vi "ARCO Reactor Read Client.vi"() -> ()   [LabVIEW 2017]
uses:
  <vilib>/OPCUA/controls/NodeIds.ctl
  <vilib>/OPCUA/controls/NodeId.ctl
  <vilib>/OPCUA/NI OPC UA Client.lvlib
panel:
  in  "stop":bool
  out "error out":errorcluster
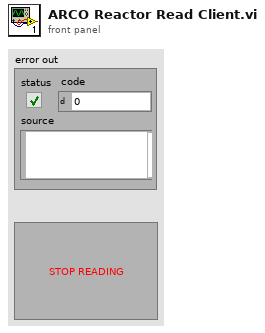
[diagram p1: front panel]
types:
  T1 = cluster{"message mode":enum16{"None", "Sign", "Sign and Encrypt"}, "security":enum16{"Basic256", "Basic128Rsa15"}}
  T2 = typedef "NodeIds.ctl" = T3[]
  T3 = typedef "NodeId.ctl" = string
  T4 = typedef "OPC UA Client Refnum.ctl" = refnum<k21>
  T5 = typedef "Subscription ID.ctl" = u32
  T6 = typedef "Subscription Data Change.ctl" = cluster{"node ID":T3, " value":variant, "timestamp":timestamp, "data type":T7, "status code":T8}
  T7 = typedef "Data Type.ctl" = u16
  T8 = typedef "OPC UA StatusCode.ctl" = u32
  T9 = cluster{"[0]":sgl, "[1]":sgl, "[2]":sgl, "[3]":sgl, "[4]":sgl, "[5]":sgl, "[6]":sgl, "[7]":sgl, "[8]":sgl, "[9]":sgl, "[10]":sgl, "[11]":sgl, "[12]":sgl, "[13]":sgl, "[14]":sgl, "[15]":sgl, "[16]":sgl, "[17]":sgl, "[18]":sgl, "[19]":sgl, "[20]":sgl, "[21]":sgl, "[22]":sgl, "[23]":sgl, "[24]":sgl, "[25]":sgl, "[26]":sgl, "[27]":sgl, "[28]":sgl, "[29]":sgl, "[30]":sgl, "[31]":sgl, "[32]":sgl, "[33]":sgl, "[34]":sgl, "[35]":sgl, "[36]":sgl, "[37]":sgl, "[38]":sgl, "[39]":sgl, "[40]":sgl, "[41]":sgl, "[42]":sgl, "[43]":sgl, "[44]":sgl, "[45]":sgl, "[46]":sgl, "[47]":sgl, "[48]":sgl, "[49]":sgl, "[50]":sgl, "[51]":sgl, "[52]":sgl, "[53]":sgl, "[54]":sgl, "[55]":sgl, "[56]":sgl}
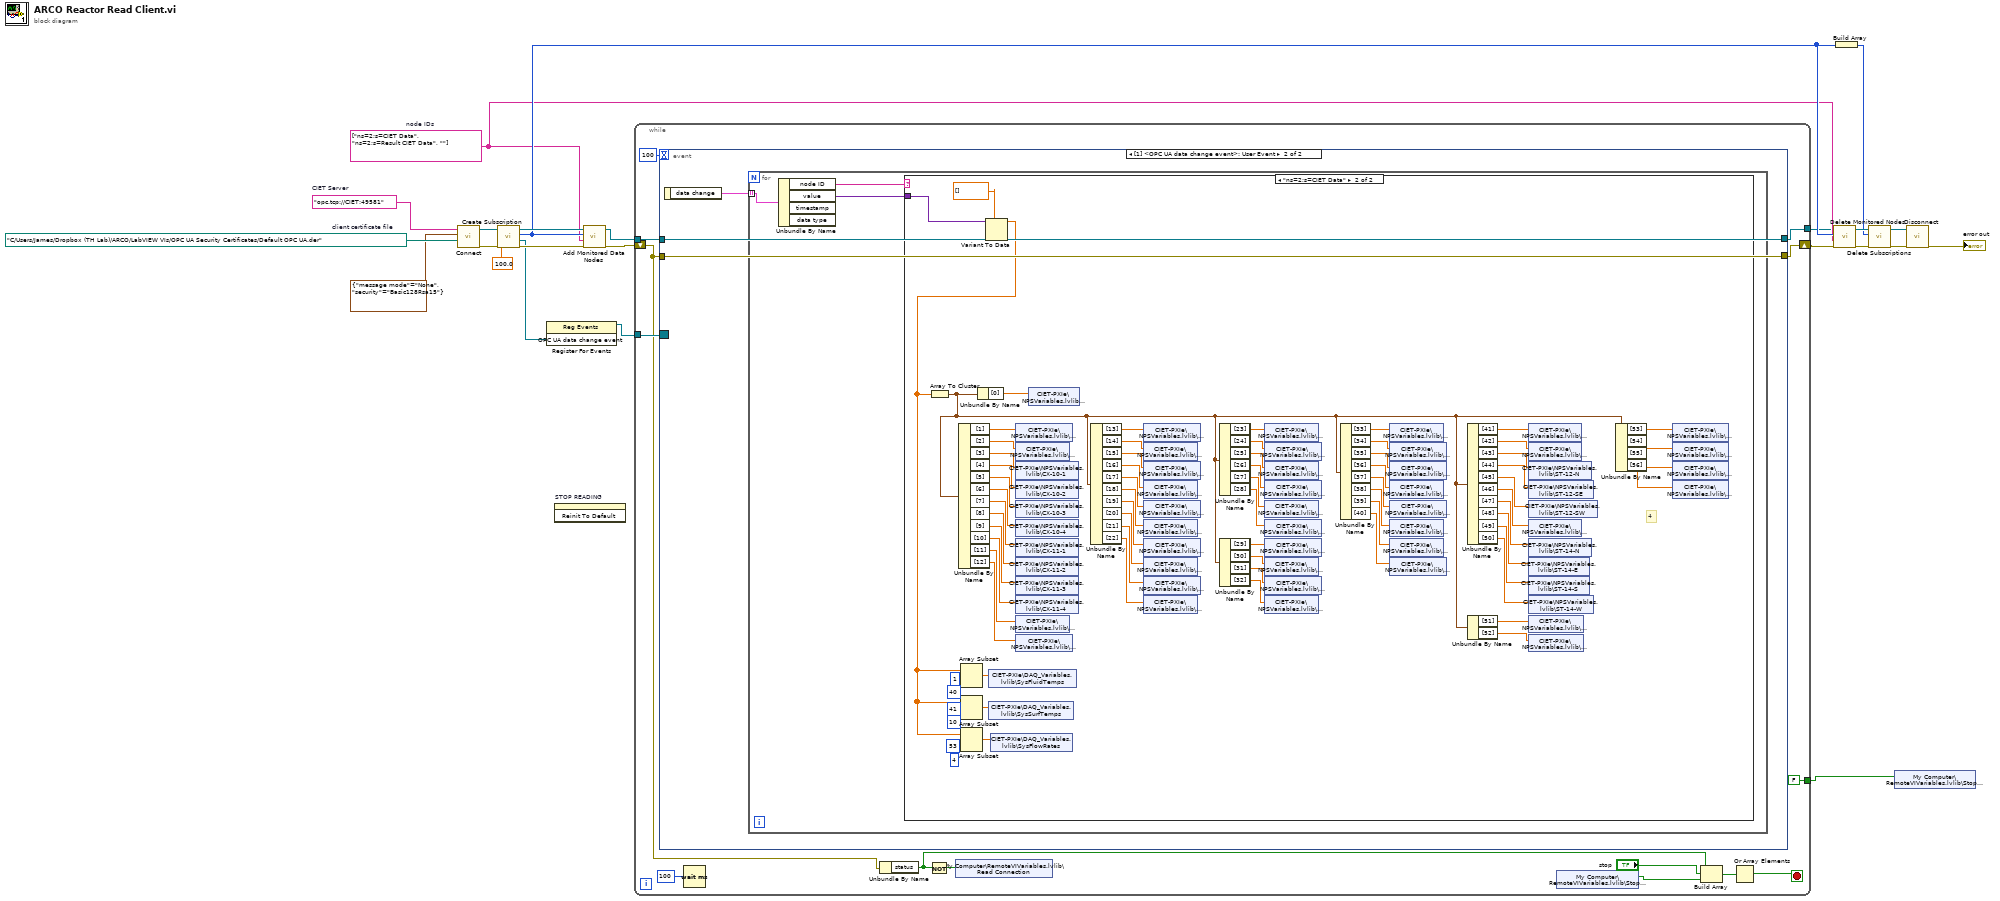
[diagram p0: block diagram]
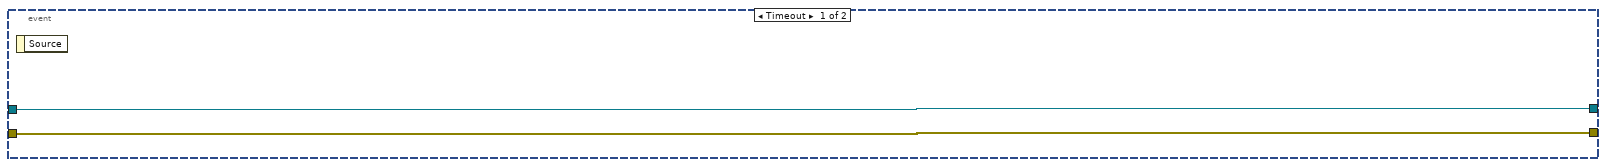
[diagram p2: hidden frame]
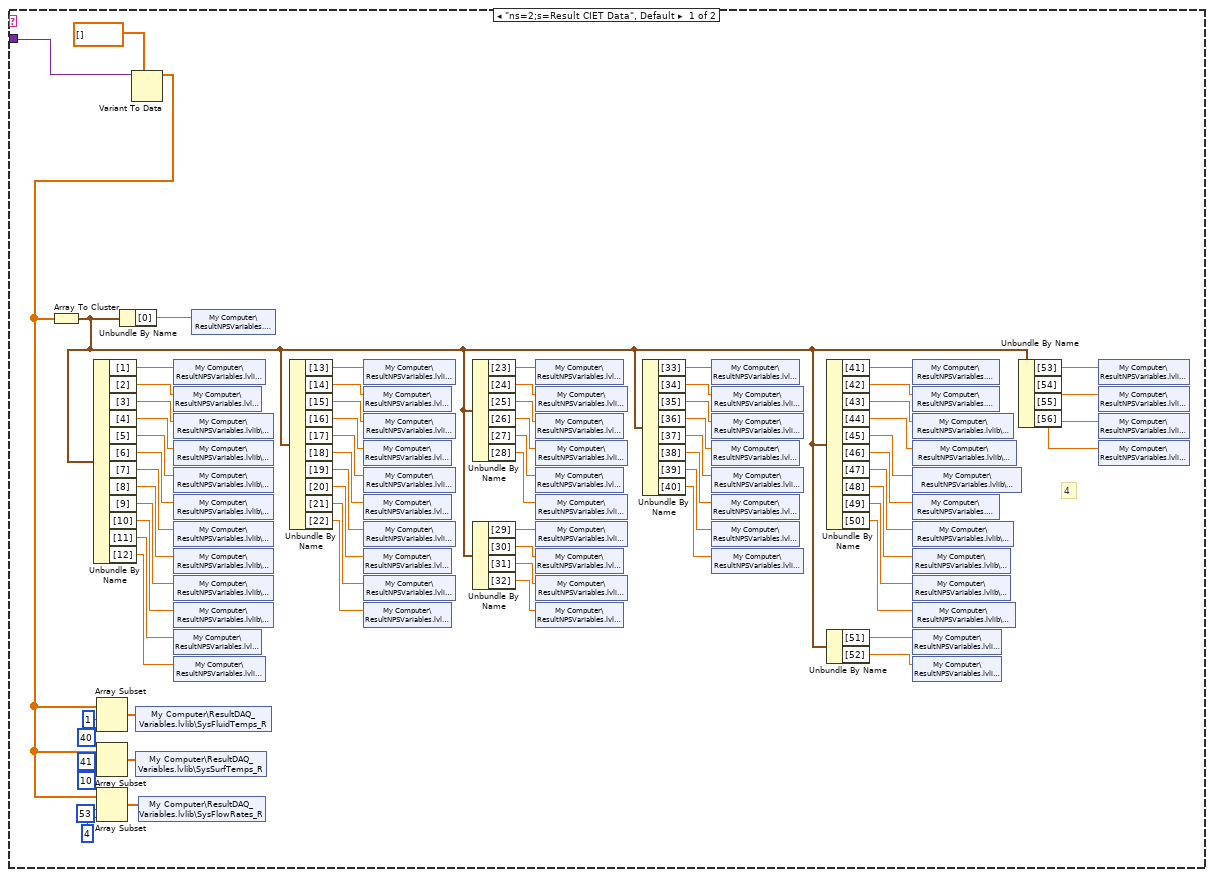
[diagram p3: hidden frame]
diagram:
  w6 = T2 ["ns=2;s=CIET Data", "ns=2;s=Result CIET Data", ""]  # node IDs
  w21 = path "C:/Users/James/Dropbox (TH Lab)/ARCO/LabVIEW VIs/OPC UA Security Certificates/Default OPC UA.der"  # client certificate file
  w22 = "opc.tcp://CIET:49581"  # CIET Server
  n1 = call <vilib>:"Connect.vi"("client certificate file"=w21, "security policy"=T1 {"message mode"=enum."None", "security"=enum."Basic128Rsa15"}, "server endpoint URL"=w22) -> ("error out"=w2:errorcluster, "OPC UA client refnum out"=w19:T4)  [unwired: 6 in, 1 out]
  n2 = call <vilib>:"Create Subscription.vi"("error in (no error)"=w2, "publishing interval (1000 ms)"=100.0, "OPC UA client refnum in"=w19) -> ("error out"=w17:errorcluster, "OPC UA data change event"=w16:refnum<user-event>, "subscription ID out"=w11:T5, "OPC UA client refnum out"=w18:T4)  [unwired: 4 in, 1 out]
  n3 = register-events(w16) -> (reference out=w9:refnum<event-registration>)  [unwired: 2 in, 1 out]
  n4 = invoke on="STOP READING" class="Bool" method="Reinit To Default"() -> ()  [unwired: 3 in, 3 out]
  n5 = call <vilib>:"Add Monitored Data Nodes.vi"("error in (no error)"=w17, "node IDs"=w6, "subscription ID in"=w11, "OPC UA client refnum in"=w18) -> ("error out"=w7:errorcluster, "OPC UA client refnum out"=w8:T4)  [unwired: 4 in, 2 out]
  n6 = while {
    tunnel: w9 -> [w37]
    tunnel: w8 -> [w36]
    tunnel: [w35] -> w5
    tunnel: [FALSE] -> w3
    shift-right: [w31] -> w1
    shift-left: w7 -> [w30]
    stop <- w29 stop-if-true
    n7 = event shown="[1] <OPC UA data change event>: User Event" {
      selector: w37 -> [_ _]
      dyn-events: _ -> [_ _]
      timeout: 100 -> [_ _]
      tunnel: w36 -> [w39 w42]
      tunnel: [w39 w42] -> w35
      tunnel: w30 -> [w38 w41]
      tunnel: [w38 w41] -> w31
      event Timeout {
        n8 = event-data() -> ()  [unwired: 1 in, 1 out]
      }
      event User Event {
        n9 = event-data() -> ("data change"=w40:T6[])  [unwired: 1 in]
        n10 = for {
          tunnel: w40 -> [w45] mode=indexing
          n11 = Unbundle By Name(w45) -> ("node ID"=w44:T3, "value"=w43:variant)  [unwired: 2 out]
          n12 = case shown="\"ns=2;s=CIET Data\"" w44 {
            tunnel: w43 -> [w48 w126]
            frame "ns=2;s=Result CIET Data", Default {
              # "4"
              n13 = Variant To Data(type=sgl[] [], Variant=w48) -> (data=w47:sgl[])  [unwired: 1 in, 1 out]
              n14 = Array To Cluster(array=w47) -> (cluster=w55:T9)
              n15 = Unbundle By Name(w55) -> ("[1]"=w56:sgl, "[2]"=w58:sgl, "[3]"=w59:sgl, "[4]"=w60:sgl, "[5]"=w61:sgl, "[6]"=w62:sgl, "[7]"=w63:sgl, "[8]"=w64:sgl, "[9]"=w65:sgl, "[10]"=w66:sgl, "[11]"=w67:sgl, "[12]"=w68:sgl)
              n16 = Array Subset(array=w47, index=1, length=40) -> (w113:sgl[])
              n17 = Array Subset(array=w47, index=41, length=10) -> (w114:sgl[])
              n18 = Array Subset(array=w47, index=53, length=4) -> (w115:sgl[])
              n19 = Unbundle By Name(w55) -> ("[0]"=w57:sgl)
              n20 = shared-variable "My Computer\\ResultDAQ_Variables.lvlib\\SysFluidTemps_R"(w113) -> ()  [unwired: 1 in, 1 out]
              n21 = shared-variable "My Computer\\ResultDAQ_Variables.lvlib\\SysSurfTemps_R"(w114) -> ()  [unwired: 1 in, 1 out]
              n22 = shared-variable "My Computer\\ResultDAQ_Variables.lvlib\\SysFlowRates_R"(w115) -> ()  [unwired: 1 in, 1 out]
              n23 = shared-variable "My Computer\\ResultNPSVariables.lvlib\\WT-10_R"(w56) -> ()  [unwired: 1 in, 1 out]
              n24 = shared-variable "My Computer\\ResultNPSVariables.lvlib\\BT-11_R"(w58) -> ()  [unwired: 1 in, 1 out]
              n25 = shared-variable "My Computer\\ResultNPSVariables.lvlib\\CX-10-1_R"(w59) -> ()  [unwired: 1 in, 1 out]
              n26 = shared-variable "My Computer\\ResultNPSVariables.lvlib\\CX-10-2_R"(w60) -> ()  [unwired: 1 in, 1 out]
              n27 = shared-variable "My Computer\\ResultNPSVariables.lvlib\\CX-10-3_R"(w61) -> ()  [unwired: 1 in, 1 out]
              n28 = shared-variable "My Computer\\ResultNPSVariables.lvlib\\CX-10-4_R"(w62) -> ()  [unwired: 1 in, 1 out]
              n29 = shared-variable "My Computer\\ResultNPSVariables.lvlib\\CX-11-1_R"(w63) -> ()  [unwired: 1 in, 1 out]
              n30 = shared-variable "My Computer\\ResultNPSVariables.lvlib\\CX-11-2_R"(w64) -> ()  [unwired: 1 in, 1 out]
              n31 = shared-variable "My Computer\\ResultNPSVariables.lvlib\\CX-11-3_R"(w65) -> ()  [unwired: 1 in, 1 out]
              n32 = shared-variable "My Computer\\ResultNPSVariables.lvlib\\CX-11-4_R"(w66) -> ()  [unwired: 1 in, 1 out]
              n33 = shared-variable "My Computer\\ResultNPSVariables.lvlib\\BT-12_R"(w67) -> ()  [unwired: 1 in, 1 out]
              n34 = shared-variable "My Computer\\ResultNPSVariables.lvlib\\WT-13_R"(w68) -> ()  [unwired: 1 in, 1 out]
              n35 = shared-variable "My Computer\\ResultNPSVariables.lvlib\\Time_R"(w57) -> ()  [unwired: 1 in, 1 out]
              n36 = Unbundle By Name(w55) -> ("[13]"=w69:sgl, "[14]"=w70:sgl, "[15]"=w71:sgl, "[16]"=w72:sgl, "[17]"=w73:sgl, "[18]"=w74:sgl, "[19]"=w75:sgl, "[20]"=w76:sgl, "[21]"=w77:sgl, "[22]"=w78:sgl)
              n37 = shared-variable "My Computer\\ResultNPSVariables.lvlib\\WT-20_R"(w69) -> ()  [unwired: 1 in, 1 out]
              n38 = shared-variable "My Computer\\ResultNPSVariables.lvlib\\BT-21_R"(w70) -> ()  [unwired: 1 in, 1 out]
              n39 = shared-variable "My Computer\\ResultNPSVariables.lvlib\\WT-22_R"(w71) -> ()  [unwired: 1 in, 1 out]
              n40 = shared-variable "My Computer\\ResultNPSVariables.lvlib\\BT-23_R"(w72) -> ()  [unwired: 1 in, 1 out]
              n41 = shared-variable "My Computer\\ResultNPSVariables.lvlib\\WT-24_R"(w73) -> ()  [unwired: 1 in, 1 out]
              n42 = shared-variable "My Computer\\ResultNPSVariables.lvlib\\BT-25_R"(w74) -> ()  [unwired: 1 in, 1 out]
              n43 = shared-variable "My Computer\\ResultNPSVariables.lvlib\\WT-26_R"(w75) -> ()  [unwired: 1 in, 1 out]
              n44 = shared-variable "My Computer\\ResultNPSVariables.lvlib\\BT-27_R"(w76) -> ()  [unwired: 1 in, 1 out]
              n45 = shared-variable "My Computer\\ResultNPSVariables.lvlib\\WT-28_R"(w77) -> ()  [unwired: 1 in, 1 out]
              n46 = shared-variable "My Computer\\ResultNPSVariables.lvlib\\BT-29_R"(w78) -> ()  [unwired: 1 in, 1 out]
              n47 = Unbundle By Name(w55) -> ("[23]"=w79:sgl, "[24]"=w80:sgl, "[25]"=w81:sgl, "[26]"=w82:sgl, "[27]"=w83:sgl, "[28]"=w84:sgl)
              n48 = Unbundle By Name(w55) -> ("[29]"=w85:sgl, "[30]"=w86:sgl, "[31]"=w87:sgl, "[32]"=w88:sgl)
              n49 = shared-variable "My Computer\\ResultNPSVariables.lvlib\\BT-30_R"(w79) -> ()  [unwired: 1 in, 1 out]
              n50 = shared-variable "My Computer\\ResultNPSVariables.lvlib\\WT-31_R"(w80) -> ()  [unwired: 1 in, 1 out]
              n51 = shared-variable "My Computer\\ResultNPSVariables.lvlib\\BT-32_R"(w81) -> ()  [unwired: 1 in, 1 out]
              n52 = shared-variable "My Computer\\ResultNPSVariables.lvlib\\WT-33_R"(w82) -> ()  [unwired: 1 in, 1 out]
              n53 = shared-variable "My Computer\\ResultNPSVariables.lvlib\\BT-34_R"(w83) -> ()  [unwired: 1 in, 1 out]
              n54 = shared-variable "My Computer\\ResultNPSVariables.lvlib\\WT-35_R"(w84) -> ()  [unwired: 1 in, 1 out]
              n55 = shared-variable "My Computer\\ResultNPSVariables.lvlib\\WT-40_R"(w85) -> ()  [unwired: 1 in, 1 out]
              n56 = shared-variable "My Computer\\ResultNPSVariables.lvlib\\BT-41_R"(w86) -> ()  [unwired: 1 in, 1 out]
              n57 = shared-variable "My Computer\\ResultNPSVariables.lvlib\\WT-42_R"(w87) -> ()  [unwired: 1 in, 1 out]
              n58 = shared-variable "My Computer\\ResultNPSVariables.lvlib\\BT-43_R"(w88) -> ()  [unwired: 1 in, 1 out]
              n59 = Unbundle By Name(w55) -> ("[33]"=w89:sgl, "[34]"=w90:sgl, "[35]"=w91:sgl, "[36]"=w92:sgl, "[37]"=w93:sgl, "[38]"=w94:sgl, "[39]"=w95:sgl, "[40]"=w96:sgl)
              n60 = shared-variable "My Computer\\ResultNPSVariables.lvlib\\BT-60_R"(w89) -> ()  [unwired: 1 in, 1 out]
              n61 = shared-variable "My Computer\\ResultNPSVariables.lvlib\\WT-61_R"(w90) -> ()  [unwired: 1 in, 1 out]
              n62 = shared-variable "My Computer\\ResultNPSVariables.lvlib\\WT-62_R"(w91) -> ()  [unwired: 1 in, 1 out]
              n63 = shared-variable "My Computer\\ResultNPSVariables.lvlib\\BT-63_R"(w92) -> ()  [unwired: 1 in, 1 out]
              n64 = shared-variable "My Computer\\ResultNPSVariables.lvlib\\WT-64_R"(w93) -> ()  [unwired: 1 in, 1 out]
              n65 = shared-variable "My Computer\\ResultNPSVariables.lvlib\\BT-65_R"(w94) -> ()  [unwired: 1 in, 1 out]
              n66 = shared-variable "My Computer\\ResultNPSVariables.lvlib\\BT-66_R"(w95) -> ()  [unwired: 1 in, 1 out]
              n67 = shared-variable "My Computer\\ResultNPSVariables.lvlib\\WT-67_R"(w96) -> ()  [unwired: 1 in, 1 out]
              n68 = Unbundle By Name(w55) -> ("[41]"=w97:sgl, "[42]"=w98:sgl, "[43]"=w99:sgl, "[44]"=w100:sgl, "[45]"=w101:sgl, "[46]"=w102:sgl, "[47]"=w103:sgl, "[48]"=w104:sgl, "[49]"=w105:sgl, "[50]"=w106:sgl)
              n69 = Unbundle By Name(w55) -> ("[51]"=w107:sgl, "[52]"=w108:sgl)
              n70 = shared-variable "My Computer\\ResultNPSVariables.lvlib\\ST-10_R"(w97) -> ()  [unwired: 1 in, 1 out]
              n71 = shared-variable "My Computer\\ResultNPSVariables.lvlib\\ST-11_R"(w98) -> ()  [unwired: 1 in, 1 out]
              n72 = shared-variable "My Computer\\ResultNPSVariables.lvlib\\ST-12-N_R"(w99) -> ()  [unwired: 1 in, 1 out]
              n73 = shared-variable "My Computer\\ResultNPSVariables.lvlib\\ST-12-SE_R"(w100) -> ()  [unwired: 1 in, 1 out]
              n74 = shared-variable "My Computer\\ResultNPSVariables.lvlib\\ST-12-SW_R"(w101) -> ()  [unwired: 1 in, 1 out]
              n75 = shared-variable "My Computer\\ResultNPSVariables.lvlib\\ST-13_R"(w102) -> ()  [unwired: 1 in, 1 out]
              n76 = shared-variable "My Computer\\ResultNPSVariables.lvlib\\ST-14-N_R"(w103) -> ()  [unwired: 1 in, 1 out]
              n77 = shared-variable "My Computer\\ResultNPSVariables.lvlib\\ST-14-E_R"(w104) -> ()  [unwired: 1 in, 1 out]
              n78 = shared-variable "My Computer\\ResultNPSVariables.lvlib\\ST-14-S_R"(w105) -> ()  [unwired: 1 in, 1 out]
              n79 = shared-variable "My Computer\\ResultNPSVariables.lvlib\\ST-14-W_R"(w106) -> ()  [unwired: 1 in, 1 out]
              n80 = shared-variable "My Computer\\ResultNPSVariables.lvlib\\AT-01_R"(w107) -> ()  [unwired: 1 in, 1 out]
              n81 = shared-variable "My Computer\\ResultNPSVariables.lvlib\\AT-02_R"(w108) -> ()  [unwired: 1 in, 1 out]
              n82 = Unbundle By Name(w55) -> ("[53]"=w109:sgl, "[54]"=w110:sgl, "[55]"=w111:sgl, "[56]"=w112:sgl)
              n83 = shared-variable "My Computer\\ResultNPSVariables.lvlib\\FM-20_R"(w109) -> ()  [unwired: 1 in, 1 out]
              n84 = shared-variable "My Computer\\ResultNPSVariables.lvlib\\FM-30_R"(w110) -> ()  [unwired: 1 in, 1 out]
              n85 = shared-variable "My Computer\\ResultNPSVariables.lvlib\\FM-40_R"(w111) -> ()  [unwired: 1 in, 1 out]
              n86 = shared-variable "My Computer\\ResultNPSVariables.lvlib\\FM-60_R"(w112) -> ()  [unwired: 1 in, 1 out]
            }
            frame "ns=2;s=CIET Data" {
              # "4"
              n87 = Variant To Data(type=sgl[] [], Variant=w126) -> (data=w123:sgl[])  [unwired: 1 in, 1 out]
              n88 = Array To Cluster(array=w123) -> (cluster=w122:T9)
              n89 = Unbundle By Name(w122) -> ("[1]"=w125:sgl, "[2]"=w128:sgl, "[3]"=w129:sgl, "[4]"=w130:sgl, "[5]"=w131:sgl, "[6]"=w132:sgl, "[7]"=w133:sgl, "[8]"=w134:sgl, "[9]"=w135:sgl, "[10]"=w136:sgl, "[11]"=w137:sgl, "[12]"=w138:sgl)
              n90 = Array Subset(array=w123, index=1, length=40) -> (w183:sgl[])
              n91 = Array Subset(array=w123, index=41, length=10) -> (w184:sgl[])
              n92 = Array Subset(array=w123, index=53, length=4) -> (w185:sgl[])
              n93 = Unbundle By Name(w122) -> ("[0]"=w127:sgl)
              n94 = shared-variable "CIET-PXIe\\DAQ_Variables.lvlib\\SysFluidTemps"(w183) -> ()  [unwired: 1 in, 1 out]
              n95 = shared-variable "CIET-PXIe\\DAQ_Variables.lvlib\\SysSurfTemps"(w184) -> ()  [unwired: 1 in, 1 out]
              n96 = shared-variable "CIET-PXIe\\DAQ_Variables.lvlib\\SysFlowRates"(w185) -> ()  [unwired: 1 in, 1 out]
              n97 = shared-variable "CIET-PXIe\\NPSVariables.lvlib\\WT-10"(w125) -> ()  [unwired: 1 in, 1 out]
              n98 = shared-variable "CIET-PXIe\\NPSVariables.lvlib\\BT-11"(w128) -> ()  [unwired: 1 in, 1 out]
              n99 = shared-variable "CIET-PXIe\\NPSVariables.lvlib\\CX-10-1"(w129) -> ()  [unwired: 1 in, 1 out]
              n100 = shared-variable "CIET-PXIe\\NPSVariables.lvlib\\CX-10-2"(w130) -> ()  [unwired: 1 in, 1 out]
              n101 = shared-variable "CIET-PXIe\\NPSVariables.lvlib\\CX-10-3"(w131) -> ()  [unwired: 1 in, 1 out]
              n102 = shared-variable "CIET-PXIe\\NPSVariables.lvlib\\CX-10-4"(w132) -> ()  [unwired: 1 in, 1 out]
              n103 = shared-variable "CIET-PXIe\\NPSVariables.lvlib\\CX-11-1"(w133) -> ()  [unwired: 1 in, 1 out]
              n104 = shared-variable "CIET-PXIe\\NPSVariables.lvlib\\CX-11-2"(w134) -> ()  [unwired: 1 in, 1 out]
              n105 = shared-variable "CIET-PXIe\\NPSVariables.lvlib\\CX-11-3"(w135) -> ()  [unwired: 1 in, 1 out]
              n106 = shared-variable "CIET-PXIe\\NPSVariables.lvlib\\CX-11-4"(w136) -> ()  [unwired: 1 in, 1 out]
              n107 = shared-variable "CIET-PXIe\\NPSVariables.lvlib\\BT-12"(w137) -> ()  [unwired: 1 in, 1 out]
              n108 = shared-variable "CIET-PXIe\\NPSVariables.lvlib\\WT-13"(w138) -> ()  [unwired: 1 in, 1 out]
              n109 = shared-variable "CIET-PXIe\\NPSVariables.lvlib\\Time"(w127) -> ()  [unwired: 1 in, 1 out]
              n110 = Unbundle By Name(w122) -> ("[13]"=w139:sgl, "[14]"=w140:sgl, "[15]"=w141:sgl, "[16]"=w142:sgl, "[17]"=w143:sgl, "[18]"=w144:sgl, "[19]"=w145:sgl, "[20]"=w146:sgl, "[21]"=w147:sgl, "[22]"=w148:sgl)
              n111 = shared-variable "CIET-PXIe\\NPSVariables.lvlib\\WT-20"(w139) -> ()  [unwired: 1 in, 1 out]
              n112 = shared-variable "CIET-PXIe\\NPSVariables.lvlib\\BT-21"(w140) -> ()  [unwired: 1 in, 1 out]
              n113 = shared-variable "CIET-PXIe\\NPSVariables.lvlib\\WT-22"(w141) -> ()  [unwired: 1 in, 1 out]
              n114 = shared-variable "CIET-PXIe\\NPSVariables.lvlib\\BT-23"(w142) -> ()  [unwired: 1 in, 1 out]
              n115 = shared-variable "CIET-PXIe\\NPSVariables.lvlib\\WT-24"(w143) -> ()  [unwired: 1 in, 1 out]
              n116 = shared-variable "CIET-PXIe\\NPSVariables.lvlib\\BT-25"(w144) -> ()  [unwired: 1 in, 1 out]
              n117 = shared-variable "CIET-PXIe\\NPSVariables.lvlib\\WT-26"(w145) -> ()  [unwired: 1 in, 1 out]
              n118 = shared-variable "CIET-PXIe\\NPSVariables.lvlib\\BT-27"(w146) -> ()  [unwired: 1 in, 1 out]
              n119 = shared-variable "CIET-PXIe\\NPSVariables.lvlib\\WT-28"(w147) -> ()  [unwired: 1 in, 1 out]
              n120 = shared-variable "CIET-PXIe\\NPSVariables.lvlib\\BT-29"(w148) -> ()  [unwired: 1 in, 1 out]
              n121 = Unbundle By Name(w122) -> ("[23]"=w149:sgl, "[24]"=w150:sgl, "[25]"=w151:sgl, "[26]"=w152:sgl, "[27]"=w153:sgl, "[28]"=w154:sgl)
              n122 = Unbundle By Name(w122) -> ("[29]"=w155:sgl, "[30]"=w156:sgl, "[31]"=w157:sgl, "[32]"=w158:sgl)
              n123 = shared-variable "CIET-PXIe\\NPSVariables.lvlib\\BT-30"(w149) -> ()  [unwired: 1 in, 1 out]
              n124 = shared-variable "CIET-PXIe\\NPSVariables.lvlib\\WT-31"(w150) -> ()  [unwired: 1 in, 1 out]
              n125 = shared-variable "CIET-PXIe\\NPSVariables.lvlib\\BT-32"(w151) -> ()  [unwired: 1 in, 1 out]
              n126 = shared-variable "CIET-PXIe\\NPSVariables.lvlib\\WT-33"(w152) -> ()  [unwired: 1 in, 1 out]
              n127 = shared-variable "CIET-PXIe\\NPSVariables.lvlib\\BT-34"(w153) -> ()  [unwired: 1 in, 1 out]
              n128 = shared-variable "CIET-PXIe\\NPSVariables.lvlib\\WT-35"(w154) -> ()  [unwired: 1 in, 1 out]
              n129 = shared-variable "CIET-PXIe\\NPSVariables.lvlib\\WT-40"(w155) -> ()  [unwired: 1 in, 1 out]
              n130 = shared-variable "CIET-PXIe\\NPSVariables.lvlib\\BT-41"(w156) -> ()  [unwired: 1 in, 1 out]
              n131 = shared-variable "CIET-PXIe\\NPSVariables.lvlib\\WT-42"(w157) -> ()  [unwired: 1 in, 1 out]
              n132 = shared-variable "CIET-PXIe\\NPSVariables.lvlib\\BT-43"(w158) -> ()  [unwired: 1 in, 1 out]
              n133 = Unbundle By Name(w122) -> ("[33]"=w159:sgl, "[34]"=w160:sgl, "[35]"=w161:sgl, "[36]"=w162:sgl, "[37]"=w163:sgl, "[38]"=w164:sgl, "[39]"=w165:sgl, "[40]"=w166:sgl)
              n134 = shared-variable "CIET-PXIe\\NPSVariables.lvlib\\BT-60"(w159) -> ()  [unwired: 1 in, 1 out]
              n135 = shared-variable "CIET-PXIe\\NPSVariables.lvlib\\WT-61"(w160) -> ()  [unwired: 1 in, 1 out]
              n136 = shared-variable "CIET-PXIe\\NPSVariables.lvlib\\WT-62"(w161) -> ()  [unwired: 1 in, 1 out]
              n137 = shared-variable "CIET-PXIe\\NPSVariables.lvlib\\BT-63"(w162) -> ()  [unwired: 1 in, 1 out]
              n138 = shared-variable "CIET-PXIe\\NPSVariables.lvlib\\WT-64"(w163) -> ()  [unwired: 1 in, 1 out]
              n139 = shared-variable "CIET-PXIe\\NPSVariables.lvlib\\BT-65"(w164) -> ()  [unwired: 1 in, 1 out]
              n140 = shared-variable "CIET-PXIe\\NPSVariables.lvlib\\BT-66"(w165) -> ()  [unwired: 1 in, 1 out]
              n141 = shared-variable "CIET-PXIe\\NPSVariables.lvlib\\WT-67"(w166) -> ()  [unwired: 1 in, 1 out]
              n142 = Unbundle By Name(w122) -> ("[41]"=w167:sgl, "[42]"=w168:sgl, "[43]"=w169:sgl, "[44]"=w170:sgl, "[45]"=w171:sgl, "[46]"=w172:sgl, "[47]"=w173:sgl, "[48]"=w174:sgl, "[49]"=w175:sgl, "[50]"=w176:sgl)
              n143 = Unbundle By Name(w122) -> ("[51]"=w177:sgl, "[52]"=w178:sgl)
              n144 = shared-variable "CIET-PXIe\\NPSVariables.lvlib\\ST-10"(w167) -> ()  [unwired: 1 in, 1 out]
              n145 = shared-variable "CIET-PXIe\\NPSVariables.lvlib\\ST-11"(w168) -> ()  [unwired: 1 in, 1 out]
              n146 = shared-variable "CIET-PXIe\\NPSVariables.lvlib\\ST-12-N"(w169) -> ()  [unwired: 1 in, 1 out]
              n147 = shared-variable "CIET-PXIe\\NPSVariables.lvlib\\ST-12-SE"(w170) -> ()  [unwired: 1 in, 1 out]
              n148 = shared-variable "CIET-PXIe\\NPSVariables.lvlib\\ST-12-SW"(w171) -> ()  [unwired: 1 in, 1 out]
              n149 = shared-variable "CIET-PXIe\\NPSVariables.lvlib\\ST-13"(w172) -> ()  [unwired: 1 in, 1 out]
              n150 = shared-variable "CIET-PXIe\\NPSVariables.lvlib\\ST-14-N"(w173) -> ()  [unwired: 1 in, 1 out]
              n151 = shared-variable "CIET-PXIe\\NPSVariables.lvlib\\ST-14-E"(w174) -> ()  [unwired: 1 in, 1 out]
              n152 = shared-variable "CIET-PXIe\\NPSVariables.lvlib\\ST-14-S"(w175) -> ()  [unwired: 1 in, 1 out]
              n153 = shared-variable "CIET-PXIe\\NPSVariables.lvlib\\ST-14-W"(w176) -> ()  [unwired: 1 in, 1 out]
              n154 = shared-variable "CIET-PXIe\\NPSVariables.lvlib\\AT-01"(w177) -> ()  [unwired: 1 in, 1 out]
              n155 = shared-variable "CIET-PXIe\\NPSVariables.lvlib\\AT-02"(w178) -> ()  [unwired: 1 in, 1 out]
              n156 = Unbundle By Name(w122) -> ("[53]"=w179:sgl, "[54]"=w180:sgl, "[55]"=w181:sgl, "[56]"=w182:sgl)
              n157 = shared-variable "CIET-PXIe\\NPSVariables.lvlib\\FM-20"(w179) -> ()  [unwired: 1 in, 1 out]
              n158 = shared-variable "CIET-PXIe\\NPSVariables.lvlib\\FM-30"(w180) -> ()  [unwired: 1 in, 1 out]
              n159 = shared-variable "CIET-PXIe\\NPSVariables.lvlib\\FM-40"(w181) -> ()  [unwired: 1 in, 1 out]
              n160 = shared-variable "CIET-PXIe\\NPSVariables.lvlib\\FM-60"(w182) -> ()  [unwired: 1 in, 1 out]
            }
          }
        }
      }
    }
    n161 = Wait (ms)(milliseconds to wait=u32 100 ("millisecond timer value")) -> ()  [unwired: 1 out]
    n162 = Unbundle By Name(w30) -> ("status"=w25:bool)
    n163 = Not(x=w25) -> (.not. x?=w32:bool)
    n164 = shared-variable "My Computer\\RemoteVIVariables.lvlib\\Read Connection"(w32) -> ()  [unwired: 1 in, 1 out]
    n165 = shared-variable "My Computer\\RemoteVIVariables.lvlib\\Stop Reading"() -> (w28:bool)  [unwired: 1 in, 1 out]
    n166 = Build Array(w25, "stop", w28) -> (w26:bool[])
    n167 = Or Array Elements(Boolean array=w26) -> (logical OR=w29:bool)
  }
  n168 = call <vilib>:"Delete Monitored Nodes.vi"("error in (no error)"=w1, "node IDs"=w6, "subscription ID in"=w11, "OPC UA client refnum in"=w5) -> ("error out"=w12:errorcluster, "OPC UA client refnum out"=w13:T4)  [unwired: 3 in, 3 out]
  n169 = Build Array(w11) -> (w10:T5[])
  n170 = call <vilib>:"Delete Subscriptions.vi"("error in (no error)"=w12, "subscription IDs"=w10, "OPC UA client refnum in"=w13) -> ("error out"=w14:errorcluster, "OPC UA client refnum out"=w15:T4)  [unwired: 6 in, 1 out]
  n171 = shared-variable "My Computer\\RemoteVIVariables.lvlib\\Stop Reading"(w3) -> ()  [unwired: 1 in, 1 out]
  n172 = call <vilib>:"Disconnect.vi"("error in (no error)"=w14, "OPC UA client refnum in"=w15) -> ("error out"=→"error out":errorcluster)  [unwired: 9 in]
